vi "3.vi"() -> ()   [LabVIEW 2021]
uses:
  22c318d8-aac9-4f54-a88f-b1e4a7437d0e.vi
panel:
  out "Array 3":string[](array[string])
  out "sum":i32
  out "Array 2":i32[](array[numeric])
  out "Array":string[](array[string])
  out "first subarray":string[](array[string])
  out "second subarray":string[](array[string])
  out "x+1":i32
  out "subarray":string[](array[string])
  out "array 2":string[][](array[string])
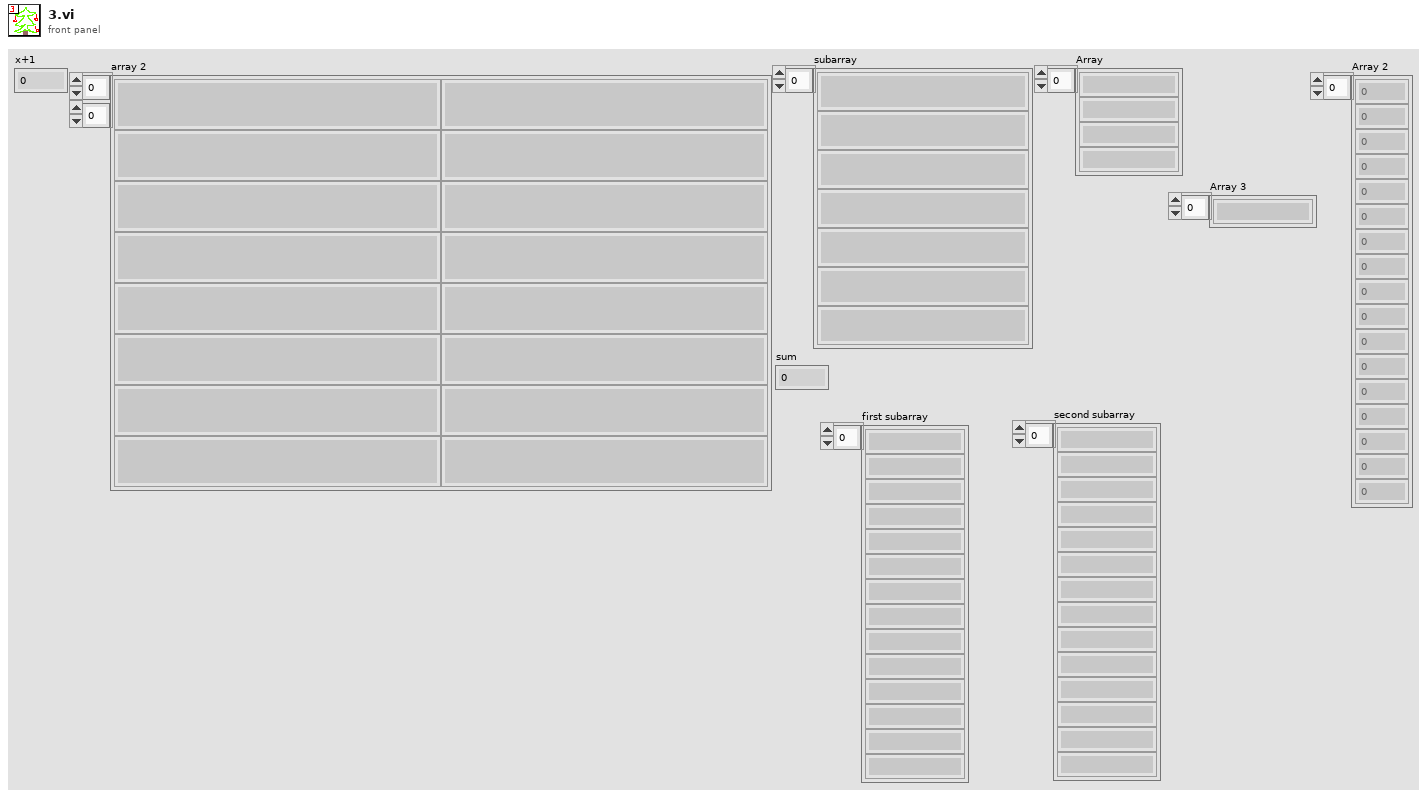
[diagram p1: front panel]
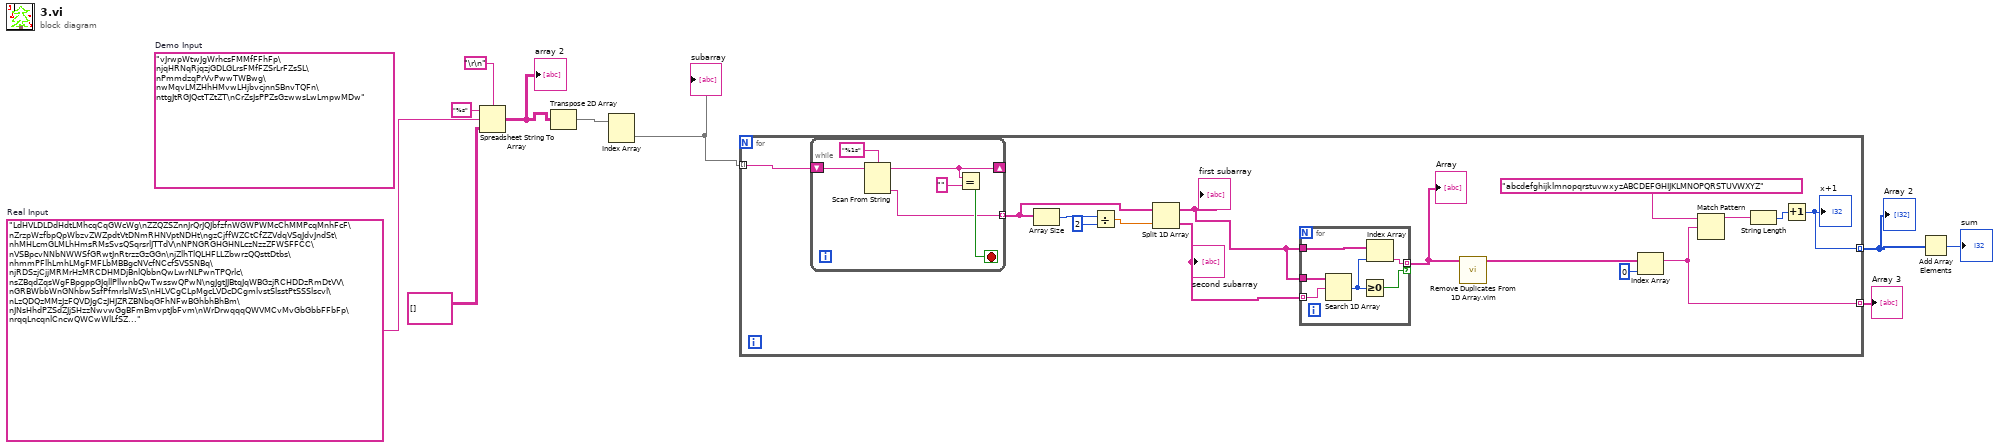
[diagram p0: block diagram]
diagram:
  w2 = "LdHVLDLDdHdtLMhcqCqGWcWg\nZZQZSZnnJrQrJQJbfzfnWGWPWMcChMMPcqMnhFcF\nZrzpWzfbpQpWbzvZWZpdtVtDNmRHNVptNDHt\ngzCjffWZCtCfZZVdqVSqJdvJndSt\nhMHLcmGLMLhHmsRMsSvsQSqrsrlJTTdV\nNPNGRGHGHNLczNzzZFWSFFCC\nVSBpcvNNbNWWSfGRwtJnRtrzzGzGGn\njZlhTlQLHFLLZbwrzQQsttDtbs\nhmmPFlhLmhLMgFMFLbMBBgcNVcfNCcfSVSSNBq\njRDSzjCjjMRMrHzMRCDHMDjBnlQbbnQwLwrNLPwnTPQrlc\nsZBqdZqsWgFBpgppGJqllPllwnbQwTwsswQPwN\ngJgtJJBtqJqWBGzjRCHDDzRmDtVV\nGRBWbbWnGNhbwSsfPfmrlslWsS\nHLVCgCLpMgcLVDcDCgmlvstSlsstPtSSSlscvl\nLzQDQzMMzJzFQVDJgCzJHJZRZBNbqGFhNFwBGhbhBhBm\nJNsHhdPZSdZJjSHzzNwvwGgBFmBmvptJbFvm\nWrDrwqqqQWVMCvMvGbGbbFFbFp\nrqqLncqnlCncwQWCwWlLfSZ..."  # Real Input
  (unwired) "vJrwpWtwJgWrhcsFMMfFFhFp\njqHRNqRjqzjGDLGLrsFMfFZSrLrFZsSL\nPmmdzqPrVvPwwTWBwg\nwMqvLMZHhHMvwLHjbvcjnnSBnvTQFn\nttgJtRGJQctTZtZT\nCrZsJsPPZsGzwwsLwLmpwMDw"  # Demo Input
  n1 = Spreadsheet String To Array(delimiter (Tab)="\r\n", format string="%s", spreadsheet string=w2, array type (2D Dbl)=string[][] []) -> (array=w7:string[][])
  "array 2" <- w7
  n2 = Transpose 2D Array(2D array=w7) -> (transposed array=w6:string[][])
  n3 = Index Array(array=w6) -> (element=w5:string[])  [unwired: 2 in]
  "subarray" <- w5
  n4 = for {
    tunnel: w5 -> [w25] mode=indexing
    tunnel: [w12] -> w4 mode=indexing
    tunnel: [w11] -> w1 mode=indexing
    n5 = while {
      shift-right: [w34] -> _
      shift-left: w25 -> [w37]
      tunnel: [w32] -> w22 mode=indexing
      stop <- w35 stop-if-true
      n6 = Scan From String(format string="%1s", input string=w37) -> (remaining string=w34:string, output 1=w32:string)  [unwired: 3 in, 2 out]
      n7 = Equal?(x=w34, y="") -> (x = y?=w35:bool)
    }
    n8 = Array Size(array=w22) -> (size(s)=w24:i32)
    n9 = Divide(x=w24, y=2) -> (x/y=w21:dbl)
    n10 = Split 1D Array(array=w22, index=w21) -> (first subarray=w20:string[], second subarray=w19:string[])
    "second subarray" <- w19
    "first subarray" <- w20
    n11 = for {
      tunnel: w19 -> [w31] mode=indexing
      tunnel: w20 -> [w28]
      tunnel: w20 -> [w30]
      tunnel: [w26] -> w18 mode=indexing if=w29
      n12 = Search 1D Array(1D array=w30, element=w31) -> (index of element=w27:i32)  [unwired: 1 in]
      n13 = Greater Or Equal To 0?(x=w27) -> (x >= 0?=w29:bool)
      n14 = Index Array(array=w28, index=w27) -> (element=w26:string)
    }
    "Array" <- w18
    n15 = call "Remove Duplicates From 1D Array.vim"("array"=w18) -> ("array with duplicates removed"=w17:string[])  [unwired: 10 in]
    n16 = Index Array(array=w17, index=0) -> (element=w11:string)
    n17 = Match Pattern(string="abcdefghijklmnopqrstuvwxyzABCDEFGHIJKLMNOPQRSTUVWXYZ" ("y"), regular expression=w11) -> (before substring=w15:string)  [unwired: 1 in, 3 out]
    n18 = String Length(string=w15) -> (length=w16:i32)
    n19 = Increment(x=w16) -> (x+1=w12:i32)
    "x+1" <- w12
  }
  "Array 2" <- w4
  "Array 3" <- w1
  n20 = Add Array Elements(numeric array=w4) -> (sum=→"sum":i32)
